vi "Get Params.vi"(8 "error in (no error)":errorcluster, 10 "Log Class":refnum<class "Build_Javier_Lopez_lib_Configuration_Filejson class.lvclass">, 11 "Module Database Manager in":refnum<class "Database Manager.lvclass">) -> (0 "error out":errorcluster, 3 "Module Database Manager out":refnum<class "Database Manager.lvclass">)   [LabVIEW 2021, in "Database Manager.lvclass"]
uses:
  Database Manager.lvclass
  <vilib>/Javier Lopez/Configuration File/Json Element/Build_Javier_Lopez_lib_Configuration_Filejson class.lvclass
  Database Manager.lvclass/Database Manager.ctl
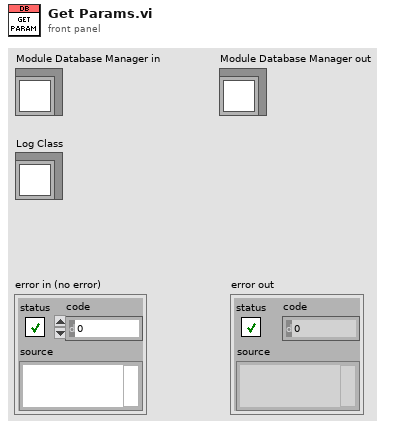
[diagram p1: front panel]
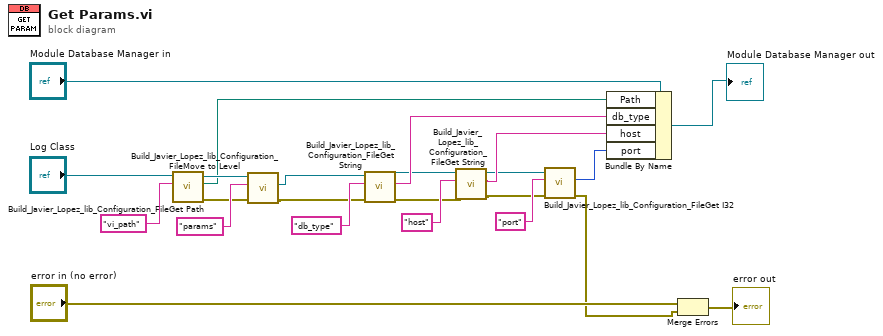
[diagram p0: block diagram]
diagram:
  n1 = call <vilib>:"Build_Javier_Lopez_lib_Configuration_FileGet Path.vi"("Name"="vi_path", "json class in"="Log Class") -> ("error out"=w16:errorcluster, "Path"=w14:path, "json class out"=w15:refnum<class "Build_Javier_Lopez_lib_Configuration_Filejson class.lvclass">)  [unwired: 7 in]
  n2 = call-dynamic "Build_Javier_Lopez_lib_Configuration_FileMove to Level.vi"("error in (no error)"=w16, "Element"="params" ("Name"), "json class in"=w15) -> ("error out"=w12:errorcluster, "New json class"=w11:refnum<class "Build_Javier_Lopez_lib_Configuration_Filejson class.lvclass">)  [unwired: 6 in, 1 out]
  n3 = call <vilib>:"Build_Javier_Lopez_lib_Configuration_FileGet String.vi"("error in (no error)"=w12, "Name"="db_type", "json class in"=w11) -> ("error out"=w8:errorcluster, "String"=w10:string, "json class out"=w7:refnum<class "Build_Javier_Lopez_lib_Configuration_Filejson class.lvclass">)  [unwired: 6 in]
  n4 = call <vilib>:"Build_Javier_Lopez_lib_Configuration_FileGet String.vi"("error in (no error)"=w8, "Name"="host", "json class in"=w7) -> ("error out"=w3:errorcluster, "String"=w6:string, "json class out"=w4:refnum<class "Build_Javier_Lopez_lib_Configuration_Filejson class.lvclass">)  [unwired: 6 in]
  n5 = call <vilib>:"Build_Javier_Lopez_lib_Configuration_FileGet I32.vi"("error in (no error)"=w3, "Name"="port", "json class in"=w4) -> ("error out"=w1:errorcluster, "I32"=w2:i32)  [unwired: 6 in, 1 out]
  n6 = Bundle By Name(cluster="Module Database Manager in", "Path"=w14, "db_type"=w10, "host"=w6, "port"=w2) -> (→"Module Database Manager out":refnum<class "Database Manager.lvclass">)
  n7 = Merge Errors("error in (no error)", w1) -> (→"error out":errorcluster)
